vi "GetBARPressures.vi"(1 "BAR Indices":i32[](array[numeric])) -> (0 "Pressures":dbl[](array[numeric]))   [LabVIEW 2011]
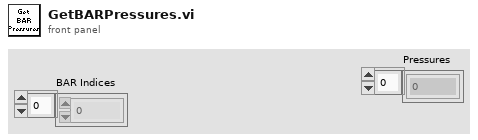
[diagram p1: front panel]
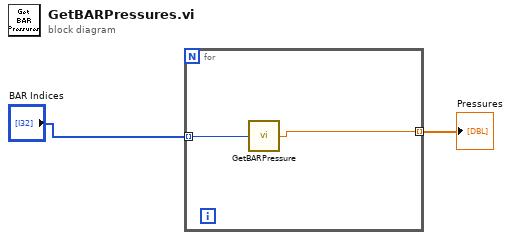
[diagram p0: block diagram]
diagram:
  n1 = for {
    tunnel: "BAR Indices" -> [w4] mode=indexing
    tunnel: [w3] -> w1 mode=indexing
    n2 = call "GetBARPressure.vi"("BAR ID Number"=w4) -> ("Pressure"=w3:dbl)
  }
  "Pressures" <- w1
